vi "Local Configuration.PCI Address.Get.vi"(8 "error in (no error)":errorcluster, 11 "GE 5565PIORC":refnum<class "GE 5565PIORC.lvclass">) -> (0 "error out":errorcluster, 2 "PCI Address":u32 format="%x", 3 "GE 5565PIORC out":refnum<class "GE 5565PIORC.lvclass">)   [LabVIEW 2016, in "GE 5565PIORC.lvclass"]
uses:
  GE 5565PIORC.lvclass
  Controls/Registers.Local Configuration.ctl
  GE 5565PIORC.lvclass/GE 5565PIORC.ctl
  <vilib>/Instr/_visa.llb/VISA Register Access Address Space.ctl
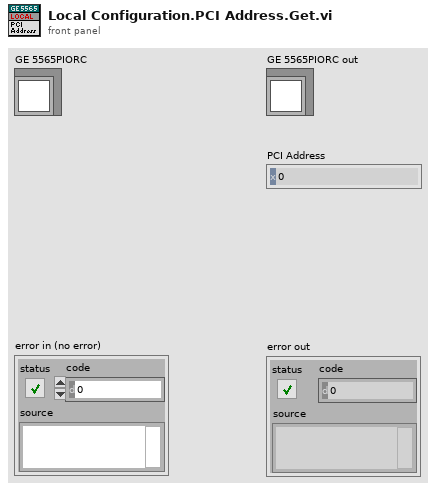
[diagram p1: front panel]
types:
  T1 = typedef "GE 5565PIORC.lvclass/Registers.Local Configuration.ctl" = enum16{"DMA Arbitration", "Interrupt Control and Status", "DMA Mode", "DMA PCI Address", "DMA Local Address", "DMA Transfer Size", "DMA Descriptor Pointer", "DMA Command/Status", "DMA PCI DAC Upper Address", "PCI PIO Address Range", "PCI PIO Base Address (Remap)"}
  T2 = typedef "VISA Register Access Address Space.ctl" = u16
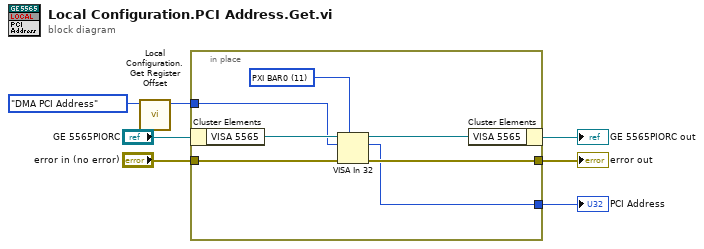
[diagram p0: block diagram]
diagram:
  n1 = call "Local Configuration.Get Register Offset.vi"("Local Configuration Register"=Registers.Local_Configuration."DMA PCI Address" ("Local Configration Register Offset")) -> ("Offset"=w1:u32)  [unwired: 10 in]
  n2 = in-place {
    in-place-border: "error in (no error)" -> [w12]
    in-place-border: [w11] -> w5
    in-place-border: [w9] -> w3
    in-place-border: w1 -> [w8]
    w10 = T2 11 items=["VXI/VME A16"=1, "VXI/VME A24"=2, "VXI/VME A32"=3, "VXI/VME A64"=4, "PXI Memory Allocations"=9, "PXI Configuration"=10, "PXI BAR0"=11, "PXI BAR1"=12, "PXI BAR2"=13, "PXI BAR3"=14, "PXI BAR4"=15, "PXI BAR5"=16] ("Address Space")
    n3 = in-place-cluster #1("GE 5565PIORC") -> ("VISA 5565"=w14:refnum<visa-resource-name>)
    n4 = VISA In 32(7:w10, 8:w12, 10:w8, 11:w14) -> (0:w11:errorcluster, 2:w9:u32, 3:w13:refnum<visa-resource-name>)
    n5 = in-place-cluster #1("VISA 5565"=w13) -> (→"GE 5565PIORC out":refnum<class "GE 5565PIORC.lvclass">)
  }
  "error out" <- w5
  "PCI Address" <- w3
